vi "PXDAC4800_LoadFileIntoRamXD48.vi"(0 "dst_offset_bytes":u32, 1 "Handle":i32, 2 "dst_length_bytes":u32, 3 "src_offset_bytes":u32, 4 "Flags":i32, 5 "src_length_bytes":u32, 6 "File_Path":string="C:\\Program Files\\Signatec\\PXDAC4800\\demo_75MHz_8bitSigned.rd8") -> (7 "Handle Out":u32, 8 "Status":i32)   [LabVIEW 2016]
uses:
  PXDAC4800.dll
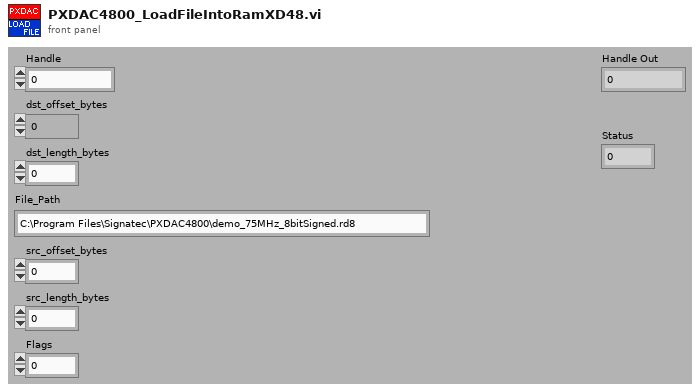
[diagram p1: front panel]
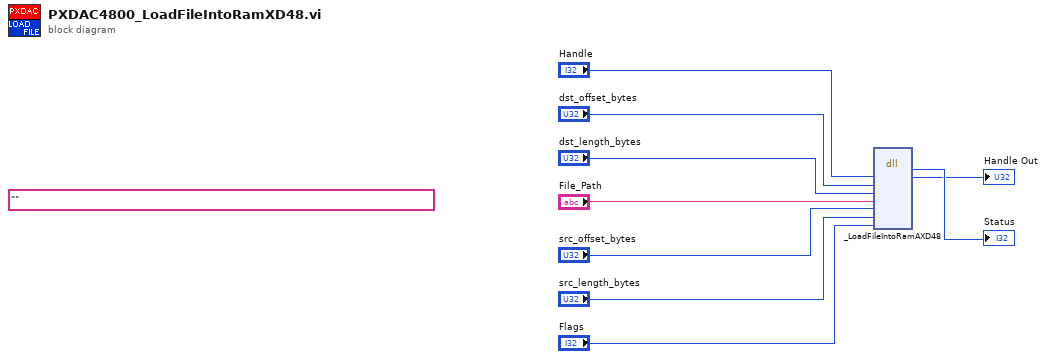
[diagram p0: block diagram]
diagram:
  (unwired) ""
  n1 = dll-call lib="PXDAC4800.dll" fn="_LoadFileIntoRamAXD48"("Handle"="Handle", "dst_offset_bytes"="dst_offset_bytes", "dst_length_bytes"="dst_length_bytes", "srcp"="File_Path", "src_offset_bytes"="src_offset_bytes", "src_length_bytes"="src_length_bytes", "flags"="Flags") -> (→"Status":i32, "Handle"=→"Handle Out":u32)  [unwired: 9 in, 2 out]
